vi "set_HR_gas.vi"(0 "As_Gas Active":bool, 1 "As_Gas Flow":dbl, 5 "As_Gas In":bool, 7 "As_Gas H2":bool, 9 "As_Gas Run":bool, 11 "As_Gas Remote":bool) -> ()   [LabVIEW 2011]
uses:
  editor_lib/Flow_Globals.vi
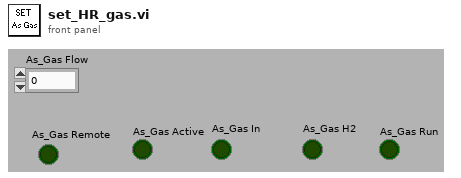
[diagram p1: front panel]
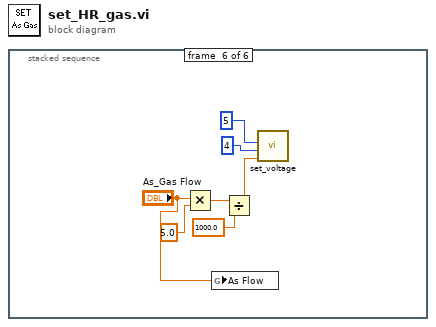
[diagram p0: block diagram]
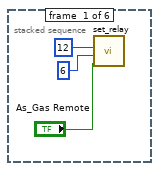
[diagram p2: hidden frame]
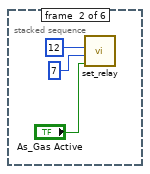
[diagram p3: hidden frame]
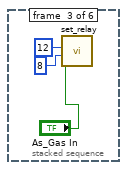
[diagram p4: hidden frame]
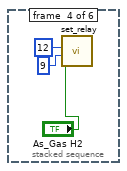
[diagram p5: hidden frame]
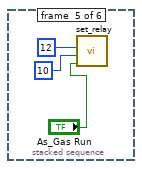
[diagram p6: hidden frame]
diagram:
  n1 = stacked-sequence {
    frame #0 {
      n2 = call "set_relay.vi"("Slot"=12, "Relay"=6, "Relay Status"="As_Gas Remote") -> ()  [unwired: 3 out]
    }
    frame #1 {
      n3 = call "set_relay.vi"("Slot"=12, "Relay"=7, "Relay Status"="As_Gas Active") -> ()  [unwired: 3 out]
    }
    frame #2 {
      n4 = call "set_relay.vi"("Slot"=12, "Relay"=8, "Relay Status"="As_Gas In") -> ()  [unwired: 1 in, 2 out]
    }
    frame #3 {
      n5 = call "set_relay.vi"("Slot"=12, "Relay"=9, "Relay Status"="As_Gas H2") -> ()  [unwired: 1 in, 2 out]
    }
    frame #4 {
      n6 = call "set_relay.vi"("Slot"=12, "Relay"=10, "Relay Status"="As_Gas Run") -> ()  [unwired: 1 in, 2 out]
    }
    frame #5 {
      n7 = Multiply(x="As_Gas Flow", y=5.0) -> (x*y=w20:dbl)
      n8 = global write "Flow_Globals.vi" "As Flow"("As_Gas Flow") -> ()
      n9 = Divide(x=w20, y=1000.0) -> (x/y=w22:dbl)
      n10 = call "set_voltage.vi"("Voltage"=w22, "Channel"=4, "Slot"=5) -> ()  [unwired: 1 in, 1 out]
    }
  }
